vi "Dual State Press Change.vi"(1 "Enable/Disable":bool, 2 "Initial":bool, 3 "Value Name":string) -> (0 "Enabled":bool)   [LabVIEW 2011]
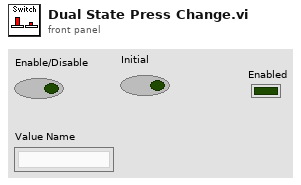
[diagram p1: front panel]
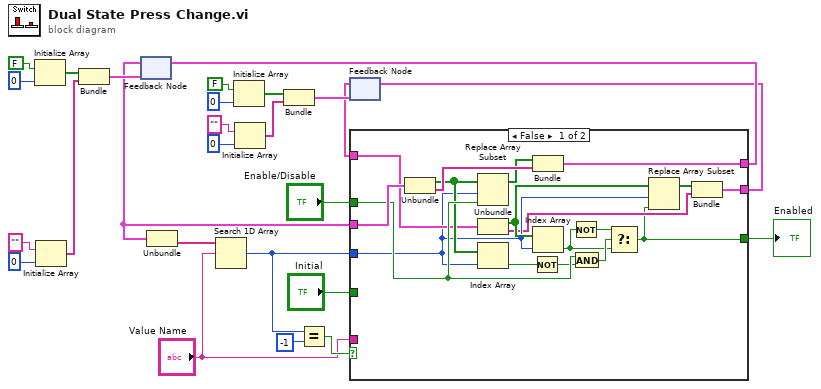
[diagram p0: block diagram]
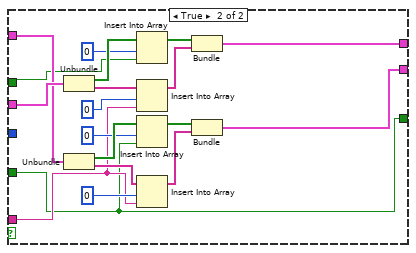
[diagram p2: hidden frame]
diagram:
  n1 = Initialize Array(FALSE, 0 ("dimension size")) -> (w26:bool[])
  n2 = Initialize Array("", 0 ("dimension size")) -> (w21:string[])
  n3 = Bundle(w26, w21) -> (w20:cluster{bool[], string[]})  [unwired: 1 in]
  n4 = feedback #1(w20) -> (w9:cluster{bool[], string[]})
  n5 = Unbundle(w9) -> (w12:string[])  [unwired: 1 out]
  n6 = Search 1D Array(1D array=w12, element="Value Name") -> (index of element=w7:i32)  [unwired: 1 in]
  n7 = Initialize Array(FALSE, 0 ("dimension size")) -> (w19:bool[])
  n8 = Initialize Array("", 0 ("dimension size")) -> (w14:string[])
  n9 = Bundle(w19, w14) -> (w13:cluster{bool[], string[]})  [unwired: 1 in]
  n10 = Equal?(x=w7, y=-1) -> (x = y?=w10:bool)
  n11 = feedback #2(w13) -> (w4:cluster{bool[], string[]})
  n12 = case shown="False" w10 {
    tunnel: w9 -> [w44 w63]
    tunnel: "Value Name" -> [_ w50]
    tunnel: w7 -> [w31 _]
    tunnel: "Enable/Disable" -> [w40 w46]
    tunnel: [w41 w56] -> w5
    tunnel: w4 -> [w36 w55]
    tunnel: [w28 w47] -> w3
    tunnel: [w27 w45] -> w2
    tunnel: "Initial" -> [_ w45]
    frame False {
      n13 = Unbundle(w44) -> (w39:bool[], w43:string[])
      n14 = Replace Array Subset(array=w39, new element=w40, index=w31) -> (w42:bool[])
      n15 = Unbundle(w36) -> (w32:bool[], w29:string[])
      n16 = Index Array(array=w39, index=w31) -> (element=w38:bool)
      n17 = Not(x=w38) -> (.not. x?=w37:bool)
      n18 = Bundle(w42, w43) -> (w41:cluster{bool[], string[]})  [unwired: 1 in]
      n19 = Index Array(array=w32, index=w31) -> (element=w33:bool)
      n20 = Not(x=w33) -> (.not. x?=w35:bool)
      n21 = And(x=w40, y=w37) -> (x .and. y?=w34:bool)
      n22 = Select(t=w35, s=w34, f=w33) -> (s? t:f=w27:bool)
      n23 = Replace Array Subset(array=w32, new element=w27, index=w31) -> (w30:bool[])
      n24 = Bundle(w30, w29) -> (w28:cluster{bool[], string[]})  [unwired: 1 in]
    }
    frame True {
      n25 = Unbundle(w63) -> (w60:bool[], w62:string[])
      n26 = Unbundle(w55) -> (w54:bool[], w53:string[])
      n27 = Insert Into Array(array=w60, index=0, new element=w46) -> (w58:bool[])
      n28 = Insert Into Array(array=w62, index=0, new element=w50) -> (w57:string[])
      n29 = Insert Into Array(array=w54, index=0, new element=w45) -> (w49:bool[])
      n30 = Insert Into Array(array=w53, index=0, new element=w50) -> (w48:string[])
      n31 = Bundle(w58, w57) -> (w56:cluster{bool[], string[]})  [unwired: 1 in]
      n32 = Bundle(w49, w48) -> (w47:cluster{bool[], string[]})  [unwired: 1 in]
    }
  }
  "Enabled" <- w2
  n33 = feedback-in #1(w5) -> ()
  n34 = feedback-in #2(w3) -> ()
